vi "CalculateDistance.vi"(1 "y0":dbl, 2 "x0":dbl, 3 "y":dbl, 4 "x":dbl) -> (0 "distance":dbl)   [LabVIEW 2020]
doc: "Calculate distance between two points as d=sqrt((x-x0)^2 + (y-y0)^2)"
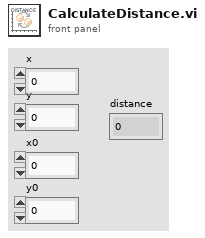
[diagram p1: front panel]
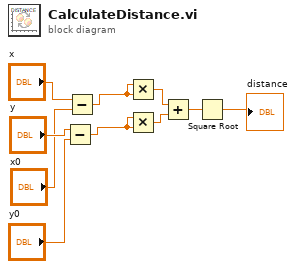
[diagram p0: block diagram]
diagram:
  n1 = Subtract(x="y", y="y0") -> (x-y=w9:dbl)
  n2 = Subtract(x="x", y="x0") -> (x-y=w8:dbl)
  n3 = Multiply(x=w8, y=w8) -> (x*y=w1:dbl)
  n4 = Multiply(x=w9, y=w9) -> (x*y=w2:dbl)
  n5 = Add(x=w1, y=w2) -> (x+y=w3:dbl)
  n6 = Square Root(x=w3) -> (sqrt(x)=→"distance":dbl)
